vi "Analog Servo FPGA Solution Rev B.vi"(9 "stop":bool) -> (1 "Clock":bool, 2 "Position Command":fxp<+,18,4>)   [LabVIEW 2012]
uses:
  <vilib>/Platform/TimedLoop/XDataNode/timing_clust.ctl
  <vilib>/Platform/TimedLoop/XDataNode/nitl_modes.ctl
  <vilib>/Platform/TimedLoop/XDataNode/wakeup.ctl
  <vilib>/rvi/Emulation/niFpgaSctlEmulationRegisterWithScheduler.vi
  <vilib>/rvi/eio/common/nirviEmuTemplateMethod_errors.vi
  <vilib>/rvi/Emulation/niFpgaSctlEmulationScheduler.vi
  <vilib>/rvi/Emulation/niFpgaSctlEmulationGetInTimedLoop.vi
  <vilib>/rvi/Emulation/niFpgaSctlEmulationGlobalWrite.vi
  <vilib>/Platform/TimedLoop/XDataNode/XDataNode.xnode
  <vilib>/eio/EIONode/EIONode.xnode
  <vilib>/Platform/TimedLoop/XDataNode/XDNodeRunTimeDep.lvlib
panel:
  out "PID Scaled Output":fxp<+/-,34,17>
  in  "Shutdown Signal":fxp<+/-,20,5>=2.5
  out "Position Feedback (Counts)":i32
  in  "Debug Command":fxp<+,14,3>
  in  "Debug?":bool
  out "Position Chart":cluster{"Position Setpoint (Deg)":i32, i32}(graph)
  in  "PID Gains":T1={"Kp"=50, "Kd"=0, "Ki"=0, "ILim"=1000, "Kv"=0, "Vff"=0, "Aff"=0, "Td"=0}
  out "Position Feedback (Counts)":i32
  in  "Reset Enc":bool
  out "Velocity (Counts/Interval)":i32
  in  "Position Setpoint (Counts)":i32
  out "Encoder B":i16(graph)
  out "Encoder A":i16(graph)
  # "Check specs for encoder \ncalibration value.  The default \nvalue is a placeholder only!"
  # "Switching into Debug mode\nwill allow you to send the\ndebug command out"
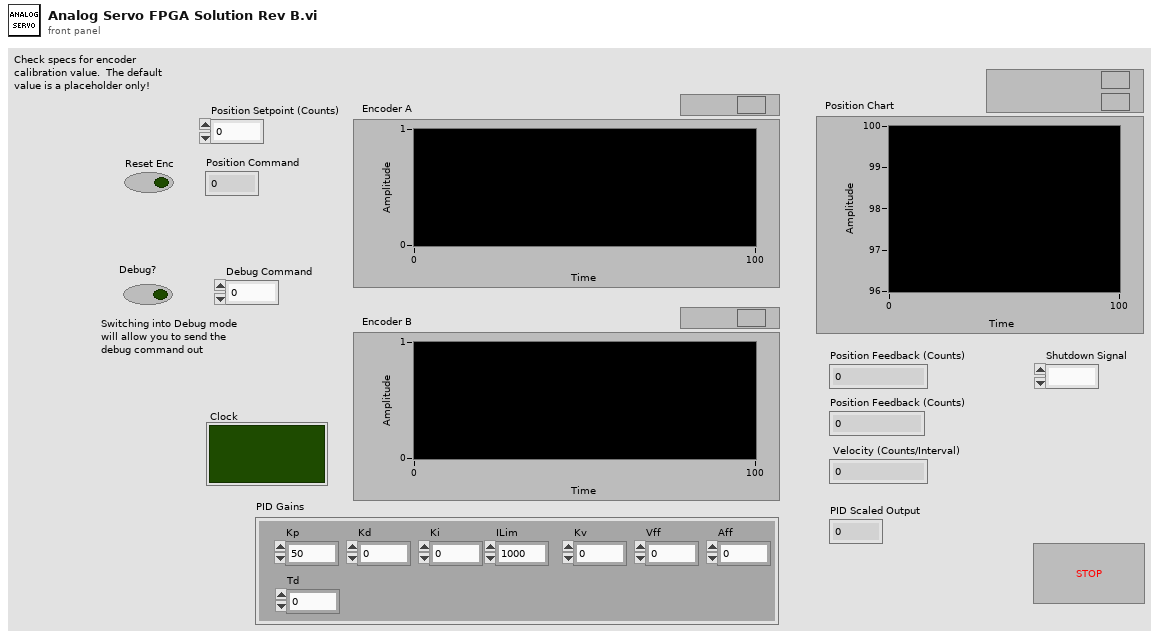
[diagram p1: front panel]
types:
  T1 = cluster{"Kp":i16, "Kd":i16, "Ki":i16, "ILim":i16, "Kv":i16, "Vff":i16, "Aff":i16, "Td":i16}
  T2 = cluster{"Position Setpoint (Counts)":i32, "Position Feedback (Counts)":i32}
  T3 = typedef "XDNodeRunTimeDep.lvlib/timing_clust.ctl" = cluster{"Expected End [f-1]":u64, "Actual End [f-1]":u64, "Finished Late? [f-1]":bool, "Expected End [i-1]":u64, "Actual End [i-1]":u64, "Finished Late? [i-1]":bool, "Expected Start [i]":u64, "Actual Start [i]":u64, "Expected Start [f]":u64, "Actual Start [f]":u64, "Source Name":string, "Structure Name":string, "Period":i64, "Deadline":i64, "Offset":i64, "Start":i64, "Priority":i32, "Timeout":i32, "Mode":T4, "Wakeup Reason":T5, "Error":errorcluster, "Source Type":string, "Secondary Source Type":string, "Global End Time":u64, "Global Start Time":u64, "Frame Duration":u64, "Iteration Duration":u64, "Assigned CPU":i32, "I/O Scan Engine Mode":u32}
  T4 = typedef "XDNodeRunTimeDep.lvlib/nitl_modes.ctl" = enum32{"No Change", "Process missed periods, maintain original phase", "Discard missed periods, maintain original phase", "Process missed periods, ignore original phase", "Discard missed periods, ignore original phase"}
  T5 = typedef "XDNodeRunTimeDep.lvlib/wakeup.ctl" = enum32{"Normal", "Aborted", "Asynchronous wakeup", "Timing source error", "Timed loop error", "Timeout"}
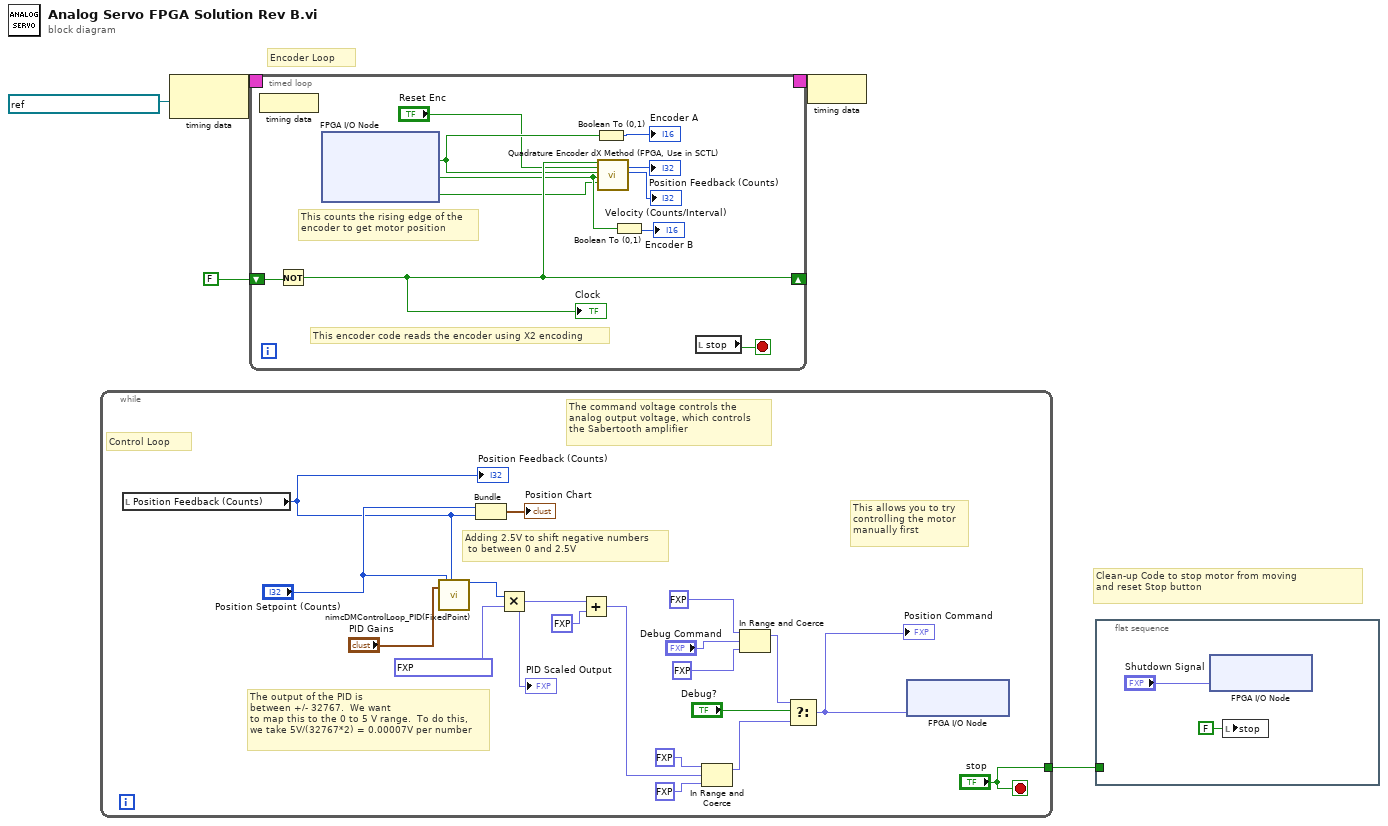
[diagram p0: block diagram]
diagram:
  # "Clean-up Code to stop motor from moving\nand reset Stop button"
  # "Encoder Loop"
  n1 = while {
    tunnel: ["stop"] -> w1
    stop <- "stop" stop-if-true
    # "Adding 2.5V to shift negative numbers\n to between 0 and 2.5V"
    # "The output of the PID is \nbetween +/- 32767.  We want\nto map this to the 0 to 5 V range.  To do this,\nwe take 5V/(32767*2) = 0.00007V per number"
    # "Control Loop"
    # "This allows you to try\ncontrolling the motor\nmanually first"
    # "The command voltage controls the \nanalog output voltage, which controls\nthe Sabertooth amplifier"
    n2 = local read "Position Feedback (Counts)"() -> (w8:i32)
    "Position Feedback (Counts)" <- w8
    n3 = call "nimcDMControlLoop_PID(FixedPoint).vi"("PID Gains"="PID Gains", "Setpoint"="Position Setpoint (Counts)", "Position Feedback"=w8) -> ("Output"=w14:i16)  [unwired: 14 in, 2 out]
    n4 = Bundle("Position Setpoint (Counts)"="Position Setpoint (Counts)", "Position Feedback (Counts)"=w8) -> (→"Position Chart":T2)  [unwired: 1 in]
    n5 = Multiply(x=w14, y=fxp<+,18,1> 7.62939453125e-05) -> (x*y=w12:fxp<+/-,34,17>)
    "PID Scaled Output" <- w12
    n6 = Add(x=w12, y=fxp<+/-,34,17> 2.5) -> (x+y=w10:fxp<+/-,18,4>)
    n7 = In Range and Coerce(upper limit=fxp<+,7,3> 5.0, x=w10, lower limit=fxp<+,7,3> 0.0 ("upper limit")) -> (coerced(x)=w9:fxp<+/-,18,4>)  [unwired: 1 out]
    n8 = In Range and Coerce(upper limit=fxp<+,7,3> 5.0, x="Debug Command", lower limit=fxp<+,1,1> 0.0) -> (coerced(x)=w19:fxp<+,14,3>)  [unwired: 1 out]
    n9 = Select(t=w19, s="Debug?", f=w9) -> (s? t:f=w15:fxp<+/-,18,4>)
    "Position Command" <- w15
    n10 = xnode "FPGA I/O Node"("Servo Drive"=w15) -> ()  [unwired: 1 in, 1 out]
  }
  n11 = node-c288(refnum<k21> "40 MHz Onboard Clock" ("Source Name")) -> (w4:T3)
  n12 = timed-loop {
    timing: w4 -> [_]
    timing-out: [_] -> w3
    shift-right: [w34] -> _
    shift-left: FALSE -> [w35]
    stop <- w25 stop-if-true
    # "This encoder code reads the encoder using X2 encoding"
    # "This counts the rising edge of the\nencoder to get motor position"
    n13 = node-c288() -> ()  [unwired: 1 in]
    n14 = Not(x=w35) -> (.not. x?=w34:bool)
    "Clock" <- w34
    n15 = xnode "FPGA I/O Node"() -> ("Encoder A"=w33:bool, "Encoder B"=w32:bool, "Encoder Index"=w29:bool)  [unwired: 3 in, 3 out]
    n16 = Boolean To (0,1)(Boolean=w33) -> (0, 1=→"Encoder A":i16)
    n17 = call "Quadrature Encoder dX Method (FPGA, Use in SCTL).vi"("Clock"=w34, "Reset Enc"="Reset Enc", "A"=w33, "B"=w32, "Z"=w29) -> ("Position (Counts)"=→"Position Feedback (Counts)":i32, "Velocity (Counts/Interval)"=→"Velocity (Counts/Interval)":i32)  [unwired: 9 in, 4 out]
    n18 = Boolean To (0,1)(Boolean=w32) -> (0, 1=→"Encoder B":i16)
    n19 = local read "stop"() -> (w25:bool)
  }
  n20 = node-c288(w3) -> ()
  n21 = flat-sequence {
    tunnel: w1 -> [_]
    frame #0 {
      n22 = xnode "FPGA I/O Node"("Servo Drive"="Shutdown Signal") -> ()  [unwired: 1 in, 1 out]
      n23 = local write "stop"(FALSE ("stop")) -> ()
    }
  }
